vi "Serialize - Text.vi"(8 "error in":errorcluster, 11 "Vaisala Data in":refnum<class "Vaisala Data.lvclass">) -> (0 "error out":errorcluster, 2 "Serialized Text":string, 3 "Vaisala Data out":refnum<class "Vaisala Data.lvclass">)   [LabVIEW 2015, in "Vaisala Library.lvlib" / "Vaisala Data.lvclass"]
uses:
  Vaisala Data.lvclass
  Vaisala Data.lvclass/Vaisala Data.ctl
  <vilib>/MSR Consulting, LLC/General Reuse/Data/Data.lvclass
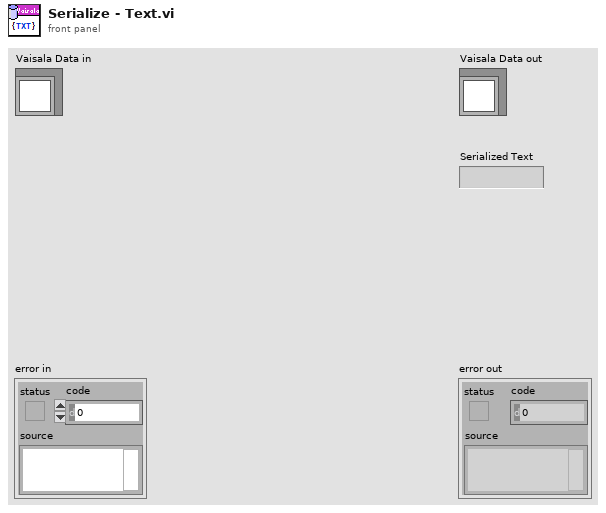
[diagram p1: front panel]
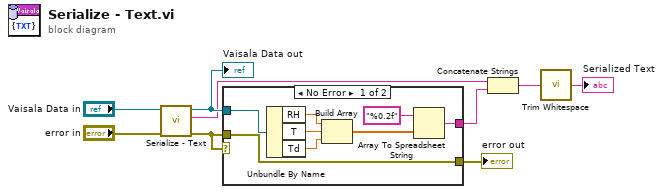
[diagram p0: block diagram]
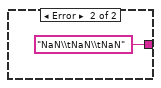
[diagram p2: hidden frame]
diagram:
  n1 = call-parent "Serialize - Text.vi"("error in"="error in", "Data in"="Vaisala Data in") -> ("error out"=w4:errorcluster, "Serialized Text"=w1:string, "Data out"=w2:refnum<class "Vaisala Data.lvclass">)  [unwired: 7 in]
  "Vaisala Data out" <- w2
  n2 = case shown="No Error" w4 {
    tunnel: w2 -> [w17 _]
    tunnel: w4 -> [w12 _]
    tunnel: [w12 _] -> w9
    tunnel: [w10 "NaN\\tNaN\\tNaN" ("spreadsheet string")] -> w7
    frame No Error {
      n3 = Unbundle By Name(w17) -> ("RH"=w16:dbl, "T"=w15:dbl, "Td"=w14:dbl)
      n4 = Build Array(w16, w15, w14) -> (w13:dbl[])
      n5 = Array To Spreadsheet String(array=w13, 3:"%0.2f" ("format string")) -> (spreadsheet string=w10:string)  [unwired: 1 in]
    }
    frame Error {
    }
  }
  "error out" <- w9
  n6 = Concatenate Strings(w1, w7) -> (w6:string)
  n7 = call <vilib>:"Trim Whitespace.vi"("string"=w6) -> ("trimmed string"=→"Serialized Text":string)  [unwired: 1 in]
